vi "VacuumCapChargingCheck.vi"(1 "Vacuum Status":T1={"Vacuum Sensors"={"TP On"=FALSE, "IG1 On"=TRUE, "IG2On"=FALSE, "IG Vac Level"=7.206095277894153e-07, "CG1 Vac Level"=7.188197481794052e-05, "CG2 Vac Level"=7.698533430214743e-05, "IG Status"=TRUE}, "In Shot Time Window"=FALSE, "IG reading meaningful"=FALSE} {"Vacuum Sensors"."CG2 Vac Level" format="%#_2e"; "Vacuum Sensors"."CG1 Vac Level" format="%#_2e"; "Vacuum Sensors"."IG Vac Level" format="%#_2e"}, 2 "Cap Charge IG Threshold":dbl=9.9e-06 min=1e-10 max=0.0001) -> (0 "IG Pressure Safe For Charging":bool)   [LabVIEW 2016]
uses:
  VacuumStatus.ctl
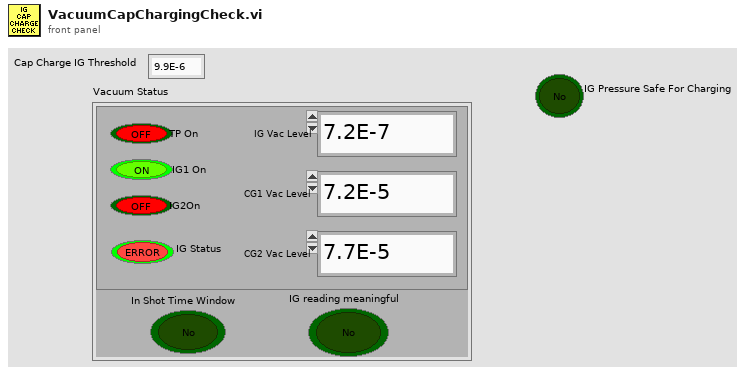
[diagram p1: front panel]
types:
  T1 = typedef "VacuumStatus.ctl" = cluster{"Vacuum Sensors":cluster{"TP On":bool, "IG1 On":bool, "IG2On":bool, "IG Vac Level":dbl, "CG1 Vac Level":dbl, "CG2 Vac Level":dbl, "IG Status":bool}, "In Shot Time Window":bool, "IG reading meaningful":bool}
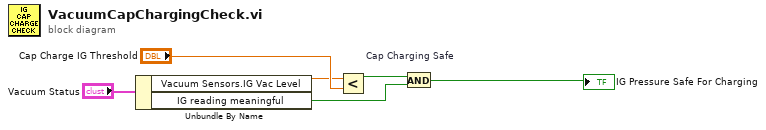
[diagram p0: block diagram]
diagram:
  n1 = Unbundle By Name("Vacuum Status") -> ("Vacuum Sensors.IG Vac Level"=w2:dbl, "IG reading meaningful"=w1:bool)
  n2 = Less?(x=w2, y="Cap Charge IG Threshold") -> (x < y?=w5:bool)
  n3 = And "Cap Charging Safe"(x=w5, y=w1) -> (x .and. y?=→"IG Pressure Safe For Charging":bool)
